vi "Which_Trav_Setup.vi"(1 "Extra Command String":string) -> (0 "Traverse Setup":string)   [LabVIEW 2010]
uses:
  Globals/Extra_Commands_Global.vi
  Globals/Trav_pos_global.vi
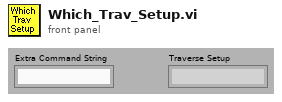
[diagram p1: front panel]
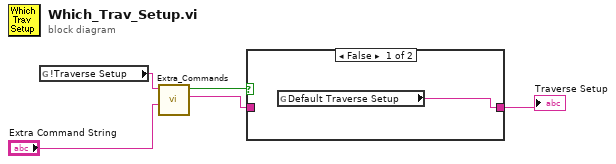
[diagram p0: block diagram]
diagram:
  n1 = global read "Extra_Commands_Global.vi" "!Traverse Setup"() -> (w2:string)
  n2 = call "Extra_Commands.vi"("String to Search"="Extra Command String", "Command"=w2) -> ("String Value"=w4:string, "Command Found"=w3:bool)  [unwired: 1 in, 3 out]
  n3 = case shown="False" w3 {
    tunnel: [w6 w7] -> w5
    tunnel: w4 -> [_ w7]
    frame False {
      n4 = global read "Trav_pos_global.vi" "Default Traverse Setup"() -> (w6:string)
    }
    frame True {
    }
  }
  "Traverse Setup" <- w5
